vi "activeXtest.vi"() -> ()   [LabVIEW 2016]
uses:
  <vilib>/Utility/NIReport.llb/NI_report.lvclass
  <vilib>/addons/_office/NI_ReportGenerationToolkit.lvlib
  <vilib>/Utility/NIReport.llb/Excel/NI_Excel.lvclass
panel:
  in  "Number of Points":i32=10
  out "cell's name":string
  in  "Select Worksheet":i32=5
  in  "start (-1, -1) 2":cluster{"row":i32, "column":i32}={"row"=-1, "column"=7}
  out "Worksheet Name":string
  out "Worksheet Names":string[](array[string])
  out "worksheets count":i32
  in  "end (-1, -1)":cluster{"row":i32, "column":i32}={"row"=-1, "column"=-1}
  in  "start (-1, -1)":cluster{"row":i32, "column":i32}={"row"=15, "column"=13}
  in  "report file path":path=path "D:/Cascade/templates/Groundwater Profiling Log_empty_1.xlsx"
  out "error out":errorcluster
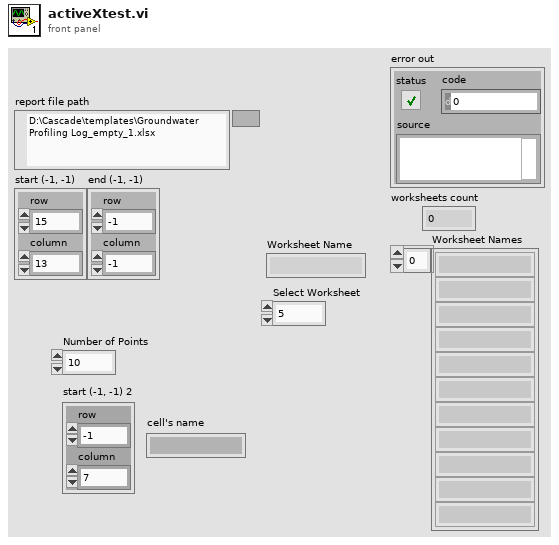
[diagram p1: front panel]
types:
  T1 = enum16{"Standard Report", "HTML", "Word", "Excel"}
  T2 = cluster{"on/off":bool, "weight":i32, "color":u32}
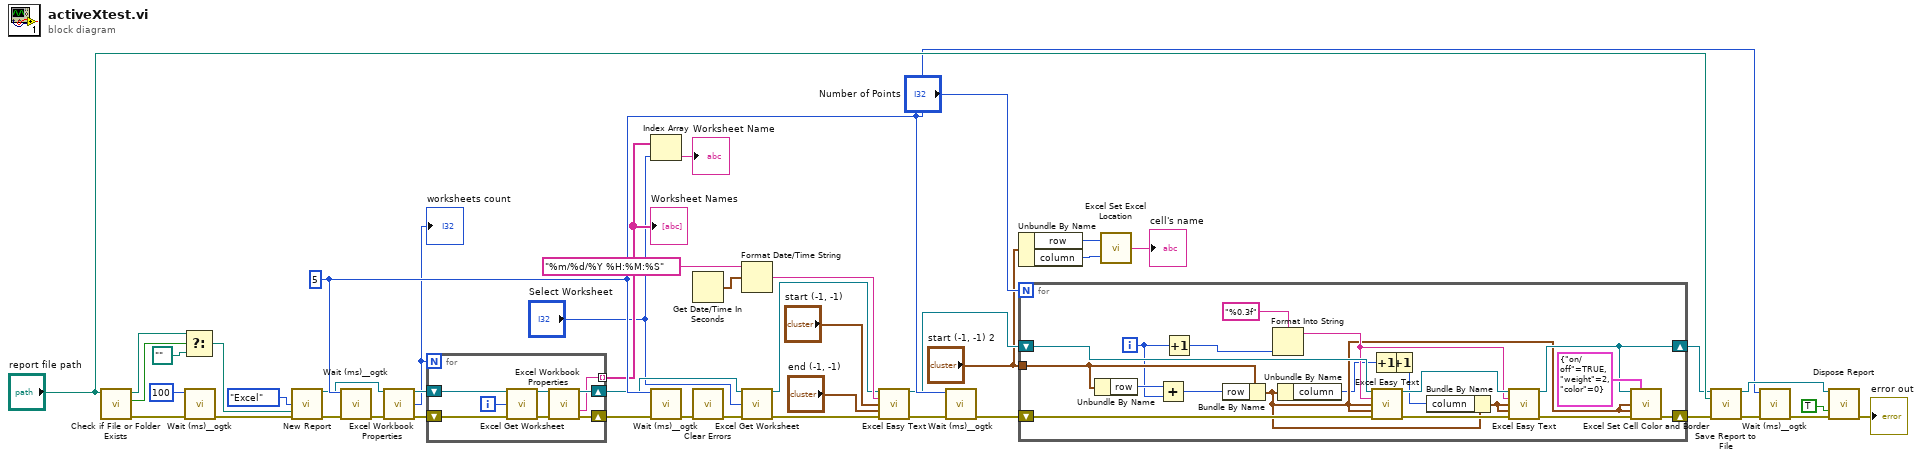
[diagram p0: block diagram]
diagram:
  w24 = u32 5 ("milliseconds to wait")
  n1 = call <vilib>:"Check if File or Folder Exists.vi"("path"="report file path") -> ("error out"=w39:errorcluster, "file or folder exists?"=w38:bool, "dup path"=w37:path)  [unwired: 8 in]
  n2 = Select(t=w37, s=w38, f=path "") -> (s? t:f=w36:path)
  n3 = call "Wait (ms)__ogtk.vi"("error in (no error)"=w39, "milliseconds to wait"=u32 100) -> ("error out"=w23:errorcluster)  [unwired: 8 in, 1 out]
  n4 = call <vilib>:"New Report.vi"("report type"=T1."Excel", "template (empty)"=w36, "error in (no error)"=w23) -> ("report out"=w21:refnum<class "NI_report.lvclass">, "error out"=w33:errorcluster)  [unwired: 11 in]
  n5 = call "Wait (ms)__ogtk.vi"("error in (no error)"=w33, "milliseconds to wait"=w24) -> ("error out"=w20:errorcluster)  [unwired: 8 in, 1 out]
  n6 = call <vilib>:"Excel Workbook Properties.vi"("report in"=w21, "error in (no error)"=w20) -> ("report out"=w18:refnum<class "NI_report.lvclass">, "worksheets count"=w17:i32, "error out"=w19:errorcluster)  [unwired: 10 in, 1 out]
  "worksheets count" <- w17
  n7 = for {
    N: w17 -> [_]
    shift-right: [w47] -> w32
    shift-left: w19 -> [w53]
    shift-right: [w48] -> w14
    shift-left: w18 -> [w52]
    tunnel: [w46] -> w6 mode=indexing
    i -> [w51]
    n8 = call <vilib>:"Excel Get Worksheet.vi"("report in"=w52, "worksheet index (0)"=w51, "error in (no error)"=w53) -> ("report out"=w49:refnum<class "NI_report.lvclass">, "error out"=w50:errorcluster)  [unwired: 11 in]
    n9 = call <vilib>:"Excel Workbook Properties.vi"("report in"=w49, "error in (no error)"=w50) -> ("report out"=w48:refnum<class "NI_report.lvclass">, "current worksheet name"=w46:string, "error out"=w47:errorcluster)  [unwired: 10 in, 1 out]
  }
  "Worksheet Names" <- w6
  n10 = Index Array(array=w6, index="Select Worksheet") -> (element=→"Worksheet Name":string)
  n11 = call "Wait (ms)__ogtk.vi"("error in (no error)"=w32, "milliseconds to wait"=w24) -> ("error out"=w26:errorcluster)  [unwired: 8 in, 1 out]
  n12 = Get Date/Time In Seconds() -> (seconds since 1Jan1904=w31:timestamp)
  n13 = call <vilib>:"Clear Errors.vi"("error in (no error)"=w26) -> ("error out"=w16:errorcluster)  [unwired: 5 in, 1 out]
  n14 = Format Date/Time String(time format string (%c)="%m/%d/%Y %H:%M:%S", seconds (now)=w31) -> (date/time string=w29:string)  [unwired: 1 in]
  n15 = call <vilib>:"Excel Get Worksheet.vi"("report in"=w14, "worksheet index (0)"="Select Worksheet", "error in (no error)"=w16) -> ("report out"=w13:refnum<class "NI_report.lvclass">, "error out"=w15:errorcluster)  [unwired: 11 in]
  n16 = call <vilib>:"Excel Easy Text.vi"("report in"=w13, "text"=w29, "start (-1, -1)"="start (-1, -1)", "end (-1, -1)"="end (-1, -1)", "error in (no error)"=w15) -> ("report out"=w10:refnum<class "NI_report.lvclass">, "error out"=w34:errorcluster)  [unwired: 6 in, 3 out]
  n17 = call "Wait (ms)__ogtk.vi"("error in (no error)"=w34, "milliseconds to wait"=w24) -> ("error out"=w12:errorcluster)  [unwired: 8 in, 1 out]
  n18 = Unbundle By Name("start (-1, -1) 2") -> ("row"=w3:i32, "column"=w2:i32)
  n19 = for {
    N: "Number of Points" -> [_]
    shift-right: [w65] -> w11
    shift-left: w12 -> [w73]
    shift-right: [w60] -> w9
    shift-left: w10 -> [w72]
    tunnel: "start (-1, -1) 2" -> [w71]
    i -> [w69]
    n20 = Unbundle By Name(w71) -> ("row"=w70:i32)
    n21 = Add(x=w70, y=w69) -> (x+y=w67:i32)
    n22 = Increment(x=w69) -> (x+1=w66:i32)
    n23 = Bundle By Name(cluster=w71, "row"=w67) -> (w58:cluster{"row":i32, "column":i32})
    n24 = Format Into String(format string="%0.3f", w66) -> (resulting string=w59:string)  [unwired: 2 in, 1 out]
    n25 = Unbundle By Name(w58) -> ("column"=w56:i32)
    n26 = Increment(x=w56) -> (x+1=w55:i32)
    n27 = call <vilib>:"Excel Easy Text.vi"("report in"=w72, "text"=w59, "start (-1, -1)"=w58, "end (-1, -1)"=w58, "error in (no error)"=w73) -> ("report out"=w61:refnum<class "NI_report.lvclass">, "error out"=w63:errorcluster)  [unwired: 6 in, 3 out]
    n28 = Increment(x=w55) -> (x+1=w54:i32)
    n29 = Bundle By Name(cluster=w58, "column"=w54) -> (w57:cluster{"row":i32, "column":i32})
    n30 = call <vilib>:"Excel Easy Text.vi"("report in"=w61, "text"=w59, "start (-1, -1)"=w57, "end (-1, -1)"=w57, "error in (no error)"=w63) -> ("report out"=w60:refnum<class "NI_report.lvclass">, "error out"=w62:errorcluster)  [unwired: 6 in, 3 out]
    n31 = call <vilib>:"Excel Set Cell Color and Border.vi"("report in"=w60, "inside border"=T2 {"on/off"=TRUE, "weight"=2, "color"=0}, "start (-1, -1)"=w58, "end (-1, -1)"=w58, "error in (no error)"=w62) -> ("error out"=w65:errorcluster)  [unwired: 9 in, 1 out]
  }
  n32 = call <vilib>:"Excel Set Excel Location.vi"("column"=w2, "row"=w3) -> ("cell's name"=→"cell's name":string)
  n33 = call-dynamic "Save Report to File.vi"("report in"=w9, "report file path"="report file path", "error in (no error)"=w11) -> ("report out"=w44:refnum<class "NI_report.lvclass">, "error out"=w43:errorcluster)  [unwired: 11 in]
  n34 = call "Wait (ms)__ogtk.vi"("error in (no error)"=w43, "milliseconds to wait"=w24) -> ("error out"=w25:errorcluster)  [unwired: 8 in, 1 out]
  n35 = call-dynamic "Dispose Report.vi"("report in"=w44, "save changes? (F)"=TRUE, "error in (no error)"=w25) -> ("error out"=→"error out":errorcluster)  [unwired: 12 in]
